vi "HFRR ADV v04.vi"() -> ()   [LabVIEW 2025] (continued)
              n1811 = String Subset(string=w2060, offset (0)=35, length (rest)=9 ("length (rest)")) -> (substring=w2085:string)
              n1812 = String Subset(string=w2060, offset (0)=55, length (rest)=9 ("length (rest)")) -> (substring=w2071:string)
              n1813 = String Subset(string=w2060, offset (0)=25, length (rest)=9 ("length (rest)")) -> (substring=w2065:string)
              n1814 = String Subset(string=w2060, offset (0)=45, length (rest)=9 ("length (rest)")) -> (substring=w2073:string)
              n1815 = String Subset(string=w2060, offset (0)=0, length (rest)=14 ("length (rest)")) -> (substring=w2088:string)
              n1816 = String Subset(string=w2060, offset (0)=15, length (rest)=9 ("length (rest)")) -> (substring=w2091:string)
              n1817 = String Subset(string=w2060, offset (0)=65, length (rest)=9 ("length (rest)")) -> (substring=w2077:string)
              n1818 = Fract/Exp String To Number(string=w2063) -> (number=w2059:dbl)  [unwired: 3 in, 1 out]
              n1819 = Fract/Exp String To Number(string=w2085) -> (number=w2083:dbl)  [unwired: 3 in, 1 out]
              n1820 = Fract/Exp String To Number(string=w2071) -> (number=w2068:dbl)  [unwired: 3 in, 1 out]
              n1821 = Fract/Exp String To Number(string=w2065) -> (number=w2064:dbl)  [unwired: 3 in, 1 out]
              n1822 = Fract/Exp String To Number(string=w2073) -> (number=w2072:dbl)  [unwired: 3 in, 1 out]
              n1823 = Fract/Exp String To Number(string=w2088) -> (number=w2084:dbl)  [unwired: 3 in, 1 out]
              n1824 = Fract/Exp String To Number(string=w2091) -> (number=w2082:dbl)  [unwired: 3 in, 1 out]
              n1825 = Fract/Exp String To Number(string=w2077) -> (number=w2080:dbl)  [unwired: 3 in, 1 out]
              n1826 = Add(x=w2080, y=0.0) -> (x+y=w2076:dbl)
            }
            n1827 = for {
              N: w1968 -> [_]
              tunnel: w1975 -> [w2023]
              tunnel: w1974 -> [w2022]
              tunnel: [w2012] -> w1928 mode=indexing
              tunnel: [w2011] -> w1921 mode=indexing
              tunnel: w1965 -> [_]
              tunnel: [w2000] -> w1926 mode=indexing
              tunnel: [w2005] -> w1923 mode=indexing
              tunnel: [w2001] -> w1913 mode=indexing
              tunnel: [w1996] -> w1888 mode=indexing
              tunnel: [w1992] -> w1869 mode=indexing
              tunnel: [w1987] -> w1829 mode=indexing
              (unwired) 1.0 ("x")
              (unwired) TRUE ("line mode (F)")
              n1828 = Read from Text File "Read File"(file (use dialog)=w2023, error in=w2022) -> (text=w1988:string)  [unwired: 2 in, 3 out]
              n1829 = local write "String 12"(w1988) -> ()
              n1830 = String Subset(string=w1988, offset (0)=85, length (rest)=9 ("length (rest)")) -> (substring=w1990:string)
              n1831 = String Subset(string=w1988, offset (0)=35, length (rest)=9 ("length (rest)")) -> (substring=w2013:string)
              n1832 = String Subset(string=w1988, offset (0)=55, length (rest)=9 ("length (rest)")) -> (substring=w1998:string)
              n1833 = String Subset(string=w1988, offset (0)=25, length (rest)=9 ("length (rest)")) -> (substring=w1994:string)
              n1834 = String Subset(string=w1988, offset (0)=45, length (rest)=9 ("length (rest)")) -> (substring=w2003:string)
              n1835 = String Subset(string=w1988, offset (0)=15, length (rest)=9 ("length (rest)")) -> (substring=w2019:string)
              n1836 = String Subset(string=w1988, offset (0)=0, length (rest)=14 ("length (rest)")) -> (substring=w2016:string)
              n1837 = String Subset(string=w1988, offset (0)=65, length (rest)=9 ("length (rest)")) -> (substring=w2006:string)
              n1838 = Fract/Exp String To Number(string=w1990) -> (number=w1987:dbl)  [unwired: 3 in, 1 out]
              n1839 = Fract/Exp String To Number(string=w2013) -> (number=w2011:dbl)  [unwired: 3 in, 1 out]
              n1840 = Fract/Exp String To Number(string=w1998) -> (number=w1996:dbl)  [unwired: 3 in, 1 out]
              n1841 = Fract/Exp String To Number(string=w1994) -> (number=w1992:dbl)  [unwired: 3 in, 1 out]
              n1842 = Fract/Exp String To Number(string=w2003) -> (number=w2001:dbl)  [unwired: 3 in, 1 out]
              n1843 = Fract/Exp String To Number(string=w2019) -> (number=w2000:dbl)  [unwired: 3 in, 1 out]
              n1844 = Fract/Exp String To Number(string=w2016) -> (number=w2012:dbl)  [unwired: 3 in, 1 out]
              n1845 = Fract/Exp String To Number(string=w2006) -> (number=w2009:dbl)  [unwired: 3 in, 1 out]
              n1846 = Add(x=w2009, y=0.0) -> (x+y=w2005:dbl)
            }
            n1847 = Delete From Array(array=w1871, index=0) -> (array with subset deleted=w1844:dbl[])  [unwired: 1 in, 1 out]
            n1848 = Delete From Array(array=w1934, index=0) -> (array with subset deleted=w1907:dbl[])  [unwired: 1 in, 1 out]
            n1849 = Delete From Array(array=w1914, index=0) -> (array with subset deleted=w1902:dbl[])  [unwired: 1 in, 1 out]
            n1850 = Delete From Array(array=w1932, index=0) -> (array with subset deleted=w1933:dbl[])  [unwired: 1 in, 1 out]
            n1851 = call-poly <vilib>:"Mean.vi"("X"=w1844) -> ("mean"=→"КОФ2 4":dbl)  [unwired: 1 out]
            n1852 = call-poly <vilib>:"Mean.vi"("X"=w1907) -> ("mean"=→"КОФ3":dbl)  [unwired: 1 out]
            n1853 = call-poly <vilib>:"Mean.vi"("X"=w1902) -> ("mean"=→"CP3":dbl)  [unwired: 1 out]
            n1854 = Delete From Array(array=w1896, index=0) -> (array with subset deleted=w1823:dbl[])  [unwired: 1 in, 1 out]
            n1855 = Delete From Array(array=w1835, index=0) -> (array with subset deleted=w1822:dbl[])  [unwired: 1 in, 1 out]
            n1856 = Delete From Array(array=w1875, index=0) -> (array with subset deleted=w1846:dbl[])  [unwired: 1 in, 1 out]
            n1857 = Delete From Array(array=w1953, index=0) -> (array with subset deleted=w1908:dbl[])  [unwired: 1 in, 1 out]
            n1858 = Delete From Array(array=w1919, index=0) -> (array with subset deleted=w1904:dbl[])  [unwired: 1 in, 1 out]
            "array w/ subset deleted" <- w1904
            n1859 = Delete From Array(array=w1950, index=0) -> (array with subset deleted=w1951:dbl[])  [unwired: 1 in, 1 out]
            n1860 = call-poly <vilib>:"Mean.vi"("X"=w1846) -> ("mean"=→"КОФ2 2":dbl)  [unwired: 1 out]
            n1861 = call-poly <vilib>:"Mean.vi"("X"=w1908) -> ("mean"=→"КОФ1":dbl)  [unwired: 1 out]
            n1862 = Bundle "Bundle"(w1823, w1822) -> (w1828:cluster{dbl[], dbl[]})  [unwired: 1 in]
            n1863 = Bundle "Bundle"(w1823, w1951) -> (w1815:cluster{dbl[], dbl[]})  [unwired: 1 in]
            n1864 = Delete From Array(array=w1830, index=0) -> (array with subset deleted=w1818:dbl[])  [unwired: 1 in, 1 out]
            n1865 = Delete From Array(array=w1831, index=0) -> (array with subset deleted=w1820:dbl[])  [unwired: 1 in, 1 out]
            n1866 = Delete From Array(array=w1941, index=0) -> (array with subset deleted=w1942:dbl[])  [unwired: 1 in, 1 out]
            n1867 = Delete From Array(array=w1829, index=0) -> (array with subset deleted=w1816:dbl[])  [unwired: 1 in, 1 out]
            n1868 = Delete From Array(array=w1923, index=0) -> (array with subset deleted=w1924:dbl[])  [unwired: 1 in, 1 out]
            n1869 = Delete From Array(array=w1948, index=0) -> (array with subset deleted=w1854:dbl[])  [unwired: 1 in, 1 out]
            n1870 = Delete From Array(array=w1894, index=0) -> (array with subset deleted=w1850:dbl[])  [unwired: 1 in, 1 out]
            n1871 = Delete From Array(array=w1930, index=0) -> (array with subset deleted=w1852:dbl[])  [unwired: 1 in, 1 out]
            n1872 = Delete From Array(array=w1890, index=0) -> (array with subset deleted=w1848:dbl[])  [unwired: 1 in, 1 out]
            n1873 = Delete From Array(array=w1939, index=0) -> (array with subset deleted=w1853:dbl[])  [unwired: 1 in, 1 out]
            n1874 = Delete From Array(array=w1892, index=0) -> (array with subset deleted=w1849:dbl[])  [unwired: 1 in, 1 out]
            n1875 = Delete From Array(array=w1873, index=0) -> (array with subset deleted=w1845:dbl[])  [unwired: 1 in, 1 out]
            n1876 = Delete From Array(array=w1917, index=0) -> (array with subset deleted=w1903:dbl[])  [unwired: 1 in, 1 out]
            n1877 = Delete From Array(array=w1944, index=0) -> (array with subset deleted=w1905:dbl[])  [unwired: 1 in, 1 out]
            n1878 = Delete From Array(array=w1921, index=0) -> (array with subset deleted=w1851:dbl[])  [unwired: 1 in, 1 out]
            n1879 = Delete From Array(array=w1888, index=0) -> (array with subset deleted=w1847:dbl[])  [unwired: 1 in, 1 out]
            n1880 = Delete From Array(array=w1869, index=0) -> (array with subset deleted=w1843:dbl[])  [unwired: 1 in, 1 out]
            n1881 = Delete From Array(array=w1913, index=0) -> (array with subset deleted=w1901:dbl[])  [unwired: 1 in, 1 out]
            n1882 = Delete From Array(array=w1926, index=0) -> (array with subset deleted=w1906:dbl[])  [unwired: 1 in, 1 out]
            n1883 = Delete From Array(array=w1936, index=0) -> (array with subset deleted=w1819:dbl[])  [unwired: 1 in, 1 out]
            n1884 = Delete From Array(array=w1946, index=0) -> (array with subset deleted=w1821:dbl[])  [unwired: 1 in, 1 out]
            n1885 = Delete From Array(array=w1928, index=0) -> (array with subset deleted=w1817:dbl[])  [unwired: 1 in, 1 out]
            n1886 = Bundle "Bundle"(w1823, w1854) -> (w1841:cluster{dbl[], dbl[]})  [unwired: 1 in]
            n1887 = Bundle "Bundle"(w1823, w1908) -> (w1842:cluster{dbl[], dbl[]})  [unwired: 1 in]
            n1888 = Bundle "Bundle"(w1854, w1850) -> (w1856:cluster{dbl[], dbl[]})  [unwired: 1 in]
            n1889 = Bundle "Bundle"(w1819, w1818) -> (w1826:cluster{dbl[], dbl[]})  [unwired: 1 in]
            n1890 = Bundle "Bundle"(w1852, w1848) -> (w1858:cluster{dbl[], dbl[]})  [unwired: 1 in]
            n1891 = Bundle "Bundle"(w1819, w1852) -> (w1962:cluster{dbl[], dbl[]})  [unwired: 1 in]
            n1892 = Bundle "Bundle"(w1819, w1848) -> (w1886:cluster{dbl[], dbl[]})  [unwired: 1 in]
            n1893 = Bundle "Bundle"(w1819, w1907) -> (w1972:cluster{dbl[], dbl[]})  [unwired: 1 in]
            n1894 = Bundle "Bundle"(w1819, w1902) -> (w1910:cluster{dbl[], dbl[]})  [unwired: 1 in]
            n1895 = Bundle "Bundle"(w1819, w1933) -> (w1957:cluster{dbl[], dbl[]})  [unwired: 1 in]
            n1896 = Bundle "Bundle"(w1853, w1849) -> (w1857:cluster{dbl[], dbl[]})  [unwired: 1 in]
            n1897 = Bundle "Bundle"(w1821, w1820) -> (w1827:cluster{dbl[], dbl[]})  [unwired: 1 in]
            n1898 = Bundle "Bundle"(w1821, w1853) -> (w1964:cluster{dbl[], dbl[]})  [unwired: 1 in]
            n1899 = Bundle "Bundle"(w1821, w1849) -> (w1887:cluster{dbl[], dbl[]})  [unwired: 1 in]
            n1900 = Bundle "Bundle"(w1821, w1903) -> (w1911:cluster{dbl[], dbl[]})  [unwired: 1 in]
            n1901 = Bundle "Bundle"(w1821, w1905) -> (w1973:cluster{dbl[], dbl[]})  [unwired: 1 in]
            n1902 = Bundle "Bundle"(w1821, w1942) -> (w1955:cluster{dbl[], dbl[]})  [unwired: 1 in]
            n1903 = Bundle "Bundle"(w1851, w1847) -> (w1859:cluster{dbl[], dbl[]})  [unwired: 1 in]
            n1904 = Bundle "Bundle"(w1817, w1816) -> (w1825:cluster{dbl[], dbl[]})  [unwired: 1 in]
            n1905 = Bundle "Bundle"(w1817, w1851) -> (w1963:cluster{dbl[], dbl[]})  [unwired: 1 in]
            n1906 = Bundle "Bundle"(w1817, w1847) -> (w1885:cluster{dbl[], dbl[]})  [unwired: 1 in]
            n1907 = Bundle "Bundle"(w1817, w1901) -> (w1909:cluster{dbl[], dbl[]})  [unwired: 1 in]
            n1908 = Bundle "Bundle"(w1817, w1906) -> (w1971:cluster{dbl[], dbl[]})  [unwired: 1 in]
            n1909 = Bundle "Bundle"(w1817, w1924) -> (w1956:cluster{dbl[], dbl[]})  [unwired: 1 in]
            n1910 = call-poly <vilib>:"Mean.vi"("X"=w1904) -> ("mean"=→"CP1":dbl)  [unwired: 1 out]
            n1911 = call-poly <vilib>:"Mean.vi"("X"=w1845) -> ("mean"=→"КОФ2 3":dbl)  [unwired: 1 out]
            n1912 = call-poly <vilib>:"Mean.vi"("X"=w1903) -> ("mean"=→"CP2":dbl)  [unwired: 1 out]
            n1913 = call-poly <vilib>:"Mean.vi"("X"=w1905) -> ("mean"=→"КОФ2":dbl)  [unwired: 1 out]
            n1914 = call-poly <vilib>:"Mean.vi"("X"=w1843) -> ("mean"=→"КОФ2 5":dbl)  [unwired: 1 out]
            n1915 = call-poly <vilib>:"Mean.vi"("X"=w1901) -> ("mean"=→"CP4":dbl)  [unwired: 1 out]
            n1916 = call-poly <vilib>:"Mean.vi"("X"=w1906) -> ("mean"=→"КОФ4":dbl)  [unwired: 1 out]
            n1917 = Bundle "Bundle"(w1823, w1850) -> (w1814:cluster{dbl[], dbl[]})  [unwired: 1 in]
            n1918 = Bundle "Bundle"(w1823, w1904) -> (w1837:cluster{dbl[], dbl[]})  [unwired: 1 in]
            n1919 = Build Array "Build Array"(w1814, w1837) -> (w1840:cluster{dbl[], dbl[]}[])
            "XY Graph 17" <- w1840
            n1920 = Build Array "Build Array"(w1828, w1827, w1826, w1825) -> (→"Frequency ( Hz )":cluster{dbl[], dbl[]}[])
            n1921 = Build Array "Build Array"(w1856, w1857, w1858, w1859) -> (→"Air Temp ( °C ) vs Humidity ( % RH )":cluster{dbl[], dbl[]}[])
            n1922 = Build Array "Build Array"(w1841, w1964, w1962, w1963) -> (→"Air Temperature  ( °C )":cluster{dbl[], dbl[]}[])
            n1923 = Build Array "Build Array"(w1814, w1887, w1886, w1885) -> (→"Humidity ( %RH )":cluster{dbl[], dbl[]}[])
            n1924 = Build Array "Build Array"(w1842, w1973, w1972, w1971) -> (→"Coefficient Of Friction":cluster{dbl[], dbl[]}[])
            n1925 = Build Array "Build Array"(w1837, w1911, w1910, w1909) -> (→"Sample Temperature ( °C )":cluster{dbl[], dbl[]}[])
            n1926 = Build Array "Build Array"(w1815, w1955, w1957, w1956) -> (→"XY Graph 13":cluster{dbl[], dbl[]}[])
            n1927 = Bundle "Bundle"(w1823, w1846) -> (w1868:cluster{dbl[], dbl[]})  [unwired: 1 in]
            n1928 = Bundle "Bundle"(w1819, w1844) -> (w1866:cluster{dbl[], dbl[]})  [unwired: 1 in]
            n1929 = Bundle "Bundle"(w1821, w1845) -> (w1867:cluster{dbl[], dbl[]})  [unwired: 1 in]
            n1930 = Bundle "Bundle"(w1817, w1843) -> (w1865:cluster{dbl[], dbl[]})  [unwired: 1 in]
            n1931 = Build Array "Build Array"(w1868, w1867, w1866, w1865) -> (→"Stroke ( mm )":cluster{dbl[], dbl[]}[])
            n1932 = local write "XY Graph 16"(w1840) -> ()
          }
          frame #2 {
          }
          frame #3 {
            n1933 = local write "Numeric 8"(0 ("Numeric 8")) -> ()
            n1934 = local write "Numeric 11"(0 ("Numeric 11")) -> ()
            n1935 = local write "Numeric 12"(0 ("Numeric 12")) -> ()
            n1936 = local write "Numeric 13"(0 ("Numeric 13")) -> ()
            n1937 = property on="OPEN" class="Bool (strict)"("Visible"=TRUE) -> ()  [unwired: 2 in, 2 out]
            n1938 = local read "String Control 2"() -> (w2140:string)
            n1939 = local read "String Control 4"() -> (w2139:string)
            n1940 = local read "String Control 6"() -> (w2138:string)
            n1941 = local read "String Control 8"() -> (w2137:string)
            n1942 = Match Pattern(string=w2140, regular expression="Samples / cycle :- ") -> (after substring=w2154:string)  [unwired: 1 in, 3 out]
            n1943 = Match Pattern(string=w2140, regular expression="Frequency :- ") -> (after substring=w2173:string)  [unwired: 1 in, 3 out]
            n1944 = Match Pattern(string=w2139, regular expression="Samples / cycle :- ") -> (after substring=w2150:string)  [unwired: 1 in, 3 out]
            n1945 = Match Pattern(string=w2139, regular expression="Frequency :- ") -> (after substring=w2168:string)  [unwired: 1 in, 3 out]
            n1946 = Match Pattern(string=w2138, regular expression="Samples / cycle :- ") -> (after substring=w2146:string)  [unwired: 1 in, 3 out]
            n1947 = Match Pattern(string=w2138, regular expression="Frequency :- ") -> (after substring=w2163:string)  [unwired: 1 in, 3 out]
            n1948 = Match Pattern(string=w2137, regular expression="Samples / cycle :- ") -> (after substring=w2142:string)  [unwired: 1 in, 3 out]
            n1949 = Match Pattern(string=w2137, regular expression="Frequency :- ") -> (after substring=w2158:string)  [unwired: 1 in, 3 out]
            n1950 = String Subset(string=w2154, length (rest)=6 ("length (rest)")) -> (substring=w2156:string)  [unwired: 1 in]
            n1951 = String Subset(string=w2173, length (rest)=9 ("length (rest)")) -> (substring=w2175:string)  [unwired: 1 in]
            n1952 = String Subset(string=w2150, length (rest)=6 ("length (rest)")) -> (substring=w2152:string)  [unwired: 1 in]
            n1953 = String Subset(string=w2168, length (rest)=9 ("length (rest)")) -> (substring=w2170:string)  [unwired: 1 in]
            n1954 = String Subset(string=w2146, length (rest)=6 ("length (rest)")) -> (substring=w2148:string)  [unwired: 1 in]
            n1955 = String Subset(string=w2163, length (rest)=9 ("length (rest)")) -> (substring=w2165:string)  [unwired: 1 in]
            n1956 = String Subset(string=w2142, length (rest)=6 ("length (rest)")) -> (substring=w2144:string)  [unwired: 1 in]
            n1957 = String Subset(string=w2158, length (rest)=9 ("length (rest)")) -> (substring=w2160:string)  [unwired: 1 in]
            n1958 = Fract/Exp String To Number(string=w2156) -> (number=w2136:dbl)  [unwired: 3 in, 1 out]
            n1959 = Fract/Exp String To Number(string=w2175) -> (number=w2176:dbl)  [unwired: 3 in, 1 out]
            n1960 = Fract/Exp String To Number(string=w2152) -> (number=w2135:dbl)  [unwired: 3 in, 1 out]
            n1961 = Fract/Exp String To Number(string=w2170) -> (number=w2171:dbl)  [unwired: 3 in, 1 out]
            n1962 = Fract/Exp String To Number(string=w2148) -> (number=w2134:dbl)  [unwired: 3 in, 1 out]
            n1963 = Fract/Exp String To Number(string=w2165) -> (number=w2166:dbl)  [unwired: 3 in, 1 out]
            n1964 = Fract/Exp String To Number(string=w2144) -> (number=w2133:dbl)  [unwired: 3 in, 1 out]
            n1965 = Fract/Exp String To Number(string=w2160) -> (number=w2161:dbl)  [unwired: 3 in, 1 out]
            n1966 = local write "sample1"(w2136) -> ()
            n1967 = local write "freq1"(w2176) -> ()
            n1968 = local write "sample2"(w2135) -> ()
            n1969 = local write "freq2"(w2171) -> ()
            n1970 = local write "sample3"(w2134) -> ()
            n1971 = local write "freq3"(w2166) -> ()
            n1972 = local write "sample4"(w2133) -> ()
            n1973 = local write "freq 4"(w2161) -> ()
          }
        }
      }
    }
    n1974 = case shown="True" w1625 {
      selector: w1625 -> [_ w1753]
      frame False {
      }
      frame True {
        n1975 = Not(x=w1753) -> (.not. x?=w1749:bool)
        n1976 = local write "service 3"(w1749) -> ()
        n1977 = local write "OPEN 6"(w1749) -> ()
        n1978 = call <vilib>:"System Exec.vi"("wait until completion? (T)"=TRUE, "command line"="C:\\LAB-IQ\\Scar View.exe") -> ("error out"=→"error out 5":errorcluster)  [unwired: 6 in, 3 out]
      }
    }
    n1979 = case shown="\"Acquire\", Default" w1636 {
      frame "Acquire", Default {
        w2649 = 0.2 ("y")
        w2654 = 1.0 ("y")
        w2655 = 0.8 ("y")
        # "Elapsed time\ncof\nstroke\nAir temp\nTemp\nHumidity"
        n1980 = disable-structure shown="Disabled" {
          frame Disabled {
            n1981 = local read "Flag"() -> (w2672:dbl)
            n1982 = local read "RUN"() -> (w2669:bool)
            n1983 = Not(x=w2669) -> (.not. x?=w2668:bool)
            n1984 = Equal?(x=w2672, y=10.0) -> (x = y?=w2670:bool)
            n1985 = And(x=w2670, y=w2668) -> (x .and. y?=w2667:bool)
            n1986 = case shown="True" w2667 {
              frame False {
              }
              frame True {
                w2673 = FALSE ("Heater Button")
                n1987 = local write "Humidity"(w2673) -> ()
                n1988 = local write "Heater Button"(w2673) -> ()
              }
            }
          }
          frame Enabled {
          }
        }
        n1989 = disable-structure shown="Disabled" {
          frame Disabled {
            n1990 = case shown="True" {
              selector: _ -> [_ _]
              frame False {
              }
              frame True {
                w2764 = TRUE ("Heater")
                n1991 = local write "Humidity"(w2764) -> ()
                n1992 = local write "Heater Button"(w2764) -> ()
                n1993 = local read "TEST STANDARD"() -> (w2767:T3)
                n1994 = local read "TEST STANDARD"() -> (w2762:T3)
                n1995 = Equal?(x=w2767, y=enum16{"ASTM D6079", "ISO 12156", "Custom"}."ISO 12156" ("Test Standard")) -> (x = y?=w2765:bool)
                n1996 = Equal?(x=w2762, y=enum16{"ASTM D6079", "ISO 12156", "Custom"}."ASTM D6079" ("Test Standard")) -> (x = y?=w2761:bool)
                n1997 = case shown="True" w2765 {
                  frame False {
                  }
                  frame True {
                    n1998 = local write "Heater"(TRUE ("Heater")) -> ()
                    n1999 = local write "airtempflg"(FALSE ("airtempflg")) -> ()
                  }
                }
                n2000 = case shown="True" w2761 {
                  frame False {
                  }
                  frame True {
                    n2001 = local write "Heater"(FALSE ("Heater")) -> ()
                    n2002 = local write "airtempflg"(TRUE ("airtempflg")) -> ()
                  }
                }
              }
            }
          }
          frame Enabled {
          }
        }
        n2003 = stacked-sequence {
          frame #0 {
            n2004 = case shown="True" "RST FF" {
              frame False {
              }
              frame True {
                w2830 = 0.0 ("X Scale.Range:Maximum")
                n2005 = property on="Frictional Force ( N )" class="WFChart (strict)"("XScale.Maximum"=600.0 ("X Scale.Range:Maximum"), "XScale.Minimum"=w2830, "YScale.Maximum"=10.0 ("Y Scale.Range:Maximum"), "YScale.Minimum"=w2830) -> ()  [unwired: 2 in, 2 out]
              }
            }
          }
          frame #1 {
            n2006 = case shown="True" "RST TEMP" {
              frame False {
              }
              frame True {
                n2007 = property on="Temperature ( Deg C )" class="WFChart (strict)"("XScale.Minimum"=0.0 ("X Scale.Range:Minimum"), "XScale.Maximum"=600.0 ("X Scale.Range:Maximum"), "YScale.Minimum"=0.0 ("Y Scale.Range:Minimum"), "YScale.Maximum"=100.0 ("Y Scale.Range:Maximum")) -> ()  [unwired: 2 in, 2 out]
              }
            }
          }
          frame #2 {
            n2008 = case shown="True" "RSTCOF" {
              frame False {
              }
              frame True {
                n2009 = property on="Coefficient of Friction" class="WFChart (strict)"("XScale.Minimum"=0.0 ("X Scale.Range:Minimum"), "XScale.Maximum"=600.0 ("X Scale.Range:Maximum"), "YScale.Maximum"=1.0 ("X Scale.Range:Minimum"), "YScale.Minimum"=0.0 ("X Scale.Range:Minimum")) -> ()  [unwired: 2 in, 2 out]
              }
            }
          }
          frame #3 {
            n2010 = case shown="True" "RSTCOF 2" {
              frame False {
              }
              frame True {
                (unwired) 100.0 ("Y Scale.Range:Maximum")
                (unwired) 0.0 ("Y Scale.Range:Minimum")
                (unwired) 600.0 ("X Scale.Range:Maximum")
                (unwired) 0.0 ("X Scale.Range:Minimum")
              }
            }
          }
          frame #4 {
            n2011 = case shown="True" "RSTCOF 3" {
              frame False {
              }
              frame True {
                n2012 = property on="Electrical Contact Resistance ( % )" class="WFChart (strict)"("XScale.Minimum"=0.0 ("X Scale.Range:Minimum"), "XScale.Maximum"=600.0 ("X Scale.Range:Maximum"), "YScale.Minimum"=0.0 ("Y Scale.Range:Minimum"), "YScale.Maximum"=100.0 ("Y Scale.Range:Maximum")) -> ()  [unwired: 2 in, 2 out]
              }
            }
          }
        }
        n2013 = disable-structure shown="Disabled" {
          frame Disabled {
            n2014 = case shown="True" {
              selector: _ -> [_ _]
              frame False {
              }
              frame True {
                n2015 = local read "zflag 2"() -> (w2731:dbl)
                n2016 = local read "yflag"() -> (w2733:dbl)
                n2017 = Equal?(x=w2733, y=2.0 ("tflag")) -> (x = y?=w2735:bool)
                n2018 = Equal?(x=w2731, y=3.0 ("tflag")) -> (x = y?=w2734:bool)
                n2019 = And(x=w2735, y=w2734) -> (x .and. y?=w2729:bool)
                n2020 = case shown="True" w2729 {
                  frame False {
                  }
                  frame True {
                    w2760 = 0.0 ("zflag")
                    n2021 = local write "zflag"(w2760) -> ()
                    n2022 = local write "zflag 2"(w2760) -> ()
                    n2023 = Delete(path (use dialog)=path "C:/LAB-IQ-NXT/WO 2449 TT.sig" ("file path (dialog if empty)")) -> (deleted path=w2759:path)  [unwired: 4 in, 2 out]
                    n2024 = Delete(path (use dialog)=path "C:/LAB-IQ-NXT/WO 2449 TRH.sig" ("file path (dialog if empty)")) -> (deleted path=w2754:path)  [unwired: 4 in, 2 out]
                    n2025 = local read "SEN.RUN HRS"() -> (w2746:dbl)
                    n2026 = local read "SENSOR TIME"() -> (w2744:dbl)
                    n2027 = call <vilib>:"compatOverwrite.vi"("overwrite (F)"=TRUE) -> ("overwrite?"=w2736:T23)
                    n2028 = call <vilib>:"compatOverwrite.vi"("overwrite (F)"=TRUE) -> ("overwrite?"=w2740:T23)
                    n2029 = local read "Total No. of Tests"() -> (w2747:dbl)
                    n2030 = Add(x=w2744, y=w2746) -> (x+y=w2745:dbl)
                    "SEN.RUN HRS" <- w2745
                    n2031 = Open/Create/Replace File(file path (use dialog)=w2759, operation (0:open)=w2736) -> (refnum out=w2737:refnum<file>, error out=w2738:errorcluster)  [unwired: 4 in, 1 out]
                    n2032 = Open/Create/Replace File(file path (use dialog)=w2754, operation (0:open)=w2740) -> (refnum out=w2741:refnum<file>, error out=w2742:errorcluster)  [unwired: 4 in, 1 out]
                    n2033 = Deny Access(4:w2738, 6:T21."deny none" ("deny mode (2)"), 7:w2737) -> (3:w2758:refnum<file>)  [unwired: 1 out]
                    n2034 = Deny Access(4:w2742, 6:T21."deny none" ("deny mode (2)"), 7:w2741) -> (3:w2750:refnum<file>)  [unwired: 1 out]
                    n2035 = Number To Decimal String(number=w2747) -> (decimal integer string=w2755:string)  [unwired: 1 in]
                    n2036 = Number To Decimal String(number=w2745) -> (decimal integer string=w2751:string)  [unwired: 1 in]
                    n2037 = Write to Binary File(file (use dialog)=w2758, data=w2755, 5:FALSE ("prepend array or string size? (T)")) -> ()  [unwired: 3 in, 3 out]
                    n2038 = Write to Binary File(file (use dialog)=w2750, data=w2751, 5:FALSE ("prepend array or string size? (T)")) -> ()  [unwired: 3 in, 3 out]
                  }
                }
              }
            }
          }
          frame Enabled {
          }
        }
        n2039 = local read "RUN"() -> (w2658:bool)
        n2040 = local read "run replace"() -> (w2662:bool)
        n2041 = local read "run replace"() -> (w2661:bool)
        n2042 = case shown="True" w2658 {
          frame False {
            n2043 = local write "run replace"(FALSE ("run replace")) -> ()
          }
          frame True {
            "run replace" <- TRUE ("run replace")
          }
        }
        n2044 = local read "RUN"() -> (w2666:bool)
        n2045 = local read "Set Temp"() -> (w2628:dbl)
        n2046 = local read "SetTemp"() -> (w2630:dbl)
        n2047 = case shown="False" w2666 {
          tunnel: [FALSE ("TEST RUNNING") TRUE ("TEST RUNNING")] -> w2665
          frame False {
            w2849 = 0.0 ("Flag")
            n2048 = local write "Elapsed time"(0.0 ("elapsedtime")) -> ()
            n2049 = local write "Time Remaining"(w2849) -> ()
            n2050 = local write "Flag"(w2849) -> ()
            n2051 = local write "Remaining Time"(w2849) -> ()
          }
          frame True {
            n2052 = local write "Flag"(10.0 ("Flag")) -> ()
          }
        }
        n2053 = case shown="False" w2662 {
          frame False {
            n2054 = local read "zflag"() -> (→"zflag 2":dbl)
            n2055 = local write "yflag"(2.0 ("tflag")) -> ()
            n2056 = local write "FLAG 4"(0.0 ("FLAG")) -> ()
          }
          frame True {
            n2057 = local write "yflag"(1.0 ("tflag")) -> ()
            n2058 = local write "zflag"(3.0 ("zflag")) -> ()
          }
        }
        n2059 = local read "acq 2"() -> (w2660:bool)
        n2060 = local read "AIR TEMP"() -> (w2623:dbl)
        n2061 = local read "Amb temp"() -> (w2627:dbl)
        n2062 = case shown="True" "Save & Continue" {
          frame False {
          }
          frame True {
            "acq 2" <- TRUE ("acq 2")
          }
        }
        n2063 = local read "Set Rh"() -> (w2629:dbl)
        n2064 = Add(x=w2630, y=w2655) -> (x+y=w2656:dbl)
        n2065 = Subtract(x=w2630, y=w2655) -> (x-y=w2657:dbl)
        n2066 = Add(x=w2628, y=w2649) -> (x+y=w2650:dbl)
        n2067 = Subtract(x=w2628, y=w2649) -> (x-y=w2651:dbl)
        n2068 = And(x=w2660, y=w2661) -> (x .and. y?=w2659:bool)
        n2069 = Greater Or Equal?(x=w2623, y=15.0) -> (x >= y?=w2624:bool)
        "powstat" <- w2624
        n2070 = local read "Humidity ( %RH )"() -> (w2626:dbl)
        n2071 = case shown="True" "Save & Continue" {
          frame False {
          }
          frame True {
            n2072 = while {
              tunnel: "0123456789abcdefghijklmnopqrstuvwxyzABCDEFGHIJKLMNOPQRSTUVWXYZ" ("string 2") -> [w2820]
              shift-right: [w2818] -> w2813
              shift-left: "" -> [w2817]
              i -> [w2827]
              stop <- w2826 stop-if-true
              n2073 = Random Number (0-1)() -> (number: 0 to 1=w2821:dbl)
              n2074 = Multiply(x=w2821, y=62.0) -> (x*y=w2823:dbl)
              n2075 = Decrement(x="Length") -> (x-1=w2816:i16)
              n2076 = To Word Integer(number=w2823) -> (16bit integer=w2824:i16)
              n2077 = String Subset(string=w2820, offset (0)=w2824, length (rest)=1 ("length (rest)")) -> (substring=w2819:string)
              n2078 = Greater Or Equal?(x=w2827, y=w2816) -> (x >= y?=w2826:bool)
              n2079 = Concatenate Strings(w2819, w2817) -> (w2818:string)
            }
            n2080 = local write "UUID"(w2813) -> ()
          }
        }
        n2081 = In Range and Coerce(upper limit=w2656, x=w2627, lower limit=w2657) -> (In Range?=w2646:bool)  [unwired: 1 out]
        n2082 = Add(x=w2629, y=w2654) -> (x+y=w2653:dbl)
        n2083 = Subtract(x=w2629, y=w2654) -> (x-y=w2652:dbl)
        n2084 = local read "TEMP"() -> (w2625:dbl)
        n2085 = case shown="True" "Save & Continue" {
          frame False {
          }
          frame True {
            n2086 = local read "Operator ID"() -> (w3129:string)
            n2087 = local read "FILE"() -> (w3135:string)
            n2088 = String Length(string=w3135) -> (length=w3133:i32)
            n2089 = String Length(string=w3129) -> (length=w3130:i32)
            n2090 = Greater?(x=w3133, y=0) -> (0:w3132:bool)
            n2091 = Greater?(x=w3130, y=0) -> (0:w3128:bool)
            n2092 = And(x=w3132, y=w3128) -> (x .and. y?=w3127:bool)
            n2093 = case shown="True" w3127 {
              frame False {
                n2094 = stacked-sequence {
                  frame #0 {
                    n2095 = One Button Dialog(message="Please Enter a File Name and Operator ID to save data !", button name ("OK")="Ok") -> ()  [unwired: 1 out]
                  }
                  frame #1 {
                    n2096 = local write "Save & Continue"(FALSE ("OK Button")) -> ()
                  }
                }
                n2097 = local write "Save & Continue"(FALSE ("OK Button")) -> ()
              }
              frame True {
                n2098 = stacked-sequence {
                  frame #0 {
                    n2099 = local read "FILE"() -> (w3141:string)
                    n2100 = call "file check.vi"("file name in"=w3141) -> ("file name out"=w3140:string)  [unwired: 9 in, 1 out]
                    n2101 = call <vilib>:"Application Directory.vi"() -> ("Application Directory"=w3151:path)
                    n2102 = Build Path(base path=w3151, name or relative path="data") -> (appended path=w3150:path)
                    n2103 = call <vilib>:"Trim Whitespace.vi"("string"=w3140) -> ("trimmed string"=w3148:string)  [unwired: 1 in]
                    n2104 = call <vilib>:"Trim Whitespace.vi"("string"=w3140) -> ("trimmed string"=w3149:string)  [unwired: 1 in]
                    n2105 = List Folder(path=w3150) -> (folder names=w3146:string[])  [unwired: 3 in, 3 out]
                    n2106 = Match Pattern(string=w3148, regular expression="_(") -> (before substring=w3145:string)  [unwired: 1 in, 3 out]
                    n2107 = for {
                      tunnel: w3146 -> [w3160] mode=indexing
                      tunnel: w3145 -> [w3158]
                      shift-right: [w3156] -> w3143
                      shift-left: bool[] [] -> [w3157]
                      n2108 = Match Pattern(string=w3160, regular expression="_(") -> (before substring=w3159:string)  [unwired: 1 in, 3 out]
                      n2109 = Equal?(x=w3159, y=w3158) -> (x = y?=w3155:bool)
                      n2110 = case shown="True" w3155 {
                        tunnel: w3155 -> [_ w3163]
                        tunnel: w3157 -> [w3162 w3165]
                        tunnel: [w3162 w3164] -> w3156
                        frame False {
                        }
                        frame True {
                          n2111 = Insert Into Array(array=w3165, new element=w3163) -> (w3164:bool[])  [unwired: 1 in]
                        }
                      }
                    }
                    n2112 = Equal?(x=w3146, y=w3145) -> (x = y?=w3154:bool[])
                    n2113 = Or Array Elements(Boolean array=w3154) -> (logical OR=w3153:bool)
                    n2114 = Array Size(array=w3143) -> (size(s)=w3142:i32)
                    n2115 = case shown="True" w3153 {
                      tunnel: w3149 -> [_ w3173]
                      tunnel: w3142 -> [_ w3166]
                      frame False {
                      }
                      frame True {
                        n2116 = Number To Decimal String(number=w3166) -> (decimal integer string=w3169:string)  [unwired: 1 in]
                        n2117 = Search/Split String(string=w3173, search string/char (-)="_(" ("regular expression")) -> (substring before match=w3171:string)  [unwired: 1 in, 2 out]
                        n2118 = Concatenate Strings(w3171, "_(" ("regular expression"), w3169, ")" ("regular expression")) -> (w3167:string)
                        n2119 = local write "FILE"(w3167) -> ()
                      }
                    }
                  }
                  frame #1 {
                    w3175 = 0.0
                    w3188 = cluster{"y":dbl, dbl, "y":dbl}[] [] ("History Data")
                    w3189 = FALSE ("Heater Button")
                    (unwired) ")!" ("string")
                    (unwired) ")" ("string")
                    w3187 = dbl[] [] ("History Data")
                    w3193 = "\r"
                    # "C:\\WinDucom\\Data\\"
                    # "C:\\LAB-IQ-NXT\\data"
                    n2120 = local write "Humidity ( %RH )"(w3175) -> ()
                    n2121 = local write "Frequency ( Hz )"(w3175) -> ()
                    n2122 = local write "Stroke 3"(w3175) -> ()
                    n2123 = local write "speedop"(0.0 ("PIDclk 2")) -> ()
                    n2124 = local write "Set Temp 2"(65.0 ("Set Temp 2")) -> ()
                    n2125 = local write "AIR TEMP"(w3175) -> ()
                    n2126 = local write "clk"(0.0 ("clk")) -> ()
                    n2127 = local write "Stroke 4"(w3175) -> ()
                    n2128 = local write "COF 2"(w3175) -> ()
                    n2129 = local write "TEMP"(w3175) -> ()
                    n2130 = local write "ecr 3"(w3175) -> ()
                    n2131 = local write "FF 3"(w3175) -> ()
                    n2132 = local write "FF 2"(w3175) -> ()
                    n2133 = property on="Humidity ( %RH )" class="WFChart (strict)"("History Data"=w3187) -> ()  [unwired: 2 in, 2 out]
                    n2134 = property on="Coefficient of Friction" class="WFChart (strict)"("History Data"=w3187) -> ()  [unwired: 2 in, 2 out]
                    n2135 = property on="Coefficient of Friction" class="WFChart (strict)"("History Data"=w3187) -> ()  [unwired: 2 in, 2 out]
                    n2136 = property on="Frictional Force ( N )" class="WFChart (strict)"("History Data"=w3187) -> ()  [unwired: 2 in, 2 out]
                    n2137 = property on="Electrical Contact Resistance ( % )" class="WFChart (strict)"("History Data"=w3187) -> ()  [unwired: 2 in, 2 out]
                    n2138 = property on="Electrical Contact Resistance ( % )" class="WFChart (strict)"("History Data"=w3187) -> ()  [unwired: 2 in, 2 out]
                    n2139 = property on="Temperature ( Deg C )" class="WFChart (strict)"("History Data"=w3187) -> ()  [unwired: 2 in, 2 out]
                    n2140 = property on="Frictional Force ( N )" class="WFChart (strict)"("History Data"=w3187) -> ()  [unwired: 2 in, 2 out]
                    n2141 = property on="Coefficient of Friction" class="WFChart (strict)"("History Data"=w3187) -> ()  [unwired: 2 in, 2 out]
                    n2142 = property on="Frictional Force ( N )" class="WFChart (strict)"("History Data"=w3187) -> ()  [unwired: 2 in, 2 out]
                    n2143 = property on="Electrical Contact Resistance ( % )" class="WFChart (strict)"("History Data"=w3187) -> ()  [unwired: 2 in, 2 out]
                    n2144 = property on="Temperature ( Deg C )" class="WFChart (strict)"("History Data"=w3187) -> ()  [unwired: 2 in, 2 out]
                    n2145 = property on="Humidity ( %RH )" class="WFChart (strict)"("History Data"=w3187) -> ()  [unwired: 2 in, 2 out]
                    n2146 = property on="Stroke ( mm )" class="WFChart (strict)"("History Data"=w3188) -> ()  [unwired: 2 in, 2 out]
                    n2147 = property on="Stroke ( mm )" class="WFChart (strict)"("History Data"=w3188) -> ()  [unwired: 2 in, 2 out]
                    n2148 = local write "Humidity"(w3189) -> ()
                    n2149 = local write "Heater Button"(w3189) -> ()
                    n2150 = local read "FILE"() -> (w3183:string)
                    n2151 = disable-structure shown="Enabled" {
                      disable-tunnel: [w3228 _] -> w3174
                      frame Enabled {
                        n2152 = local read "NORMAL LOAD"() -> (w3228:dbl)
                      }
                      frame Disabled {
                      }
                    }
                    n2153 = call "file check.vi"("file name in"=w3183) -> ("error out"=w3186:errorcluster, "file name out"=w3180:string)  [unwired: 9 in]
                    n2154 = call "FILE PATH CREATION.vi"("error in"=w3186, "FILE NAME :"=w3180) -> ("FILE OUT"=w3179:path)  [unwired: 8 in, 1 out]
                    n2155 = Concatenate Strings(w3180, ".dgf" ("Substring")) -> (w3185:string)
                    n2156 = Concatenate Strings(w3180, ".duf" ("Substring")) -> (w3181:string)
                    n2157 = Multiply(x=w3174, y=1.0) -> (x*y=w3207:dbl)
                    n2158 = Build Path(base path=w3179, name or relative path=w3185) -> (appended path=w3178:path)
                    n2159 = Build Path(base path=w3179, name or relative path=w3181) -> (appended path=w3177:path)
                    n2160 = Number To Fractional String(number=w3207, width (-)=i16 5, precision (6)=i16 2) -> (F-format string=w3215:string)  [unwired: 1 in]
                    n2161 = local read "Fuel Discription :"() -> (w3203:string)
                    n2162 = local read "Batch Ref Num :"() -> (w3191:string)
                    n2163 = Get Date/Time String(date format (0)=enum16{"short", "long", "abbreviated"}."short") -> (date string=w3226:string, time string=w3223:string)  [unwired: 2 in]
                    n2164 = local read "Remarks :"() -> (w3202:string)
                    n2165 = Concatenate Strings("Load :- " ("Substring"), w3215, " grams ," ("Substring")) -> (w3214:string)
                    n2166 = local read "String 41"() -> (w3194:string)
                    n2167 = Concatenate Strings(w3203) -> (w3204:string)
                    n2168 = Concatenate Strings(w3191) -> (w3190:string)
                    n2169 = Concatenate Strings("tested by") -> (w3198:string)
                    n2170 = Concatenate Strings("(" ("Substring"), w3226, ")" ("Substring"), w3223) -> (w3196:string)
                    "concatenated string" <- w3196
                    n2171 = Concatenate Strings(w3202, "," ("string")) -> (w3201:string)
                    n2172 = Concatenate Strings("  TIME;      COF;       STROKE;     AIR TEMP;  TEMP;  HUMIDITY;  ECR; PID-OUT; FREQUENCY" ("Substring"), "\r") -> (w3210:string)
                    n2173 = Concatenate Strings(w3194, w3193, "Fuel Discription :-" ("Substring"), w3204, w3193, w3214, w3193, "Batch Ref Num :-" ("Substring"), w3190, w3193, " Remarks :- " ("Substring"), w3201, w3193, " Date :- " ("Substring"), w3196, w3193, "Tested By :-" ("Substring"), w3198) -> (w3208:string)
                    "REMARKS" <- w3208
                    n2174 = call <vilib>:"Write Characters To File.vi"("append to file? (new file:F)"=FALSE, "character string"=w3210, "file path (dialog if empty)"=w3178) -> ()  [unwired: 2 in, 1 out]
                    n2175 = call <vilib>:"Write Characters To File.vi"("append to file? (new file:F)"=FALSE, "character string"=w3208, "file path (dialog if empty)"=w3177) -> ()  [unwired: 2 in, 1 out]
                  }
                  frame #2 {
                    n2176 = local write "Cycles elapsed"(0 ("Cycles elapsed")) -> ()
                    n2177 = local write "cyclecount"(0 ("cyclecount")) -> ()
                    n2178 = local write "Save & Continue"(FALSE ("OK")) -> ()
                    n2179 = local write "autostrtflg"(TRUE ("autostrtflg")) -> ()
                    n2180 = local write "Save"(FALSE ("Save")) -> ()
                    n2181 = Get Date/Time In Seconds() -> (seconds since 1Jan1904=w3233:timestamp)
                    n2182 = To Double Precision Float(number=w3233) -> (double precision float=w3232:dbl)
                    n2183 = local write "acq timer"(w3232) -> ()
                    n2184 = One Button Dialog(message="Please ensure sample is mounted properly and machine is ready in all aspects for testing !", button name ("OK")="Ok") -> ()  [unwired: 1 out]
                  }
                  frame #3 {
                    n2185 = stacked-sequence {
                      frame #0 {
                        n2186 = local write "Main Dashboard Buttons"(T1."Dashboard" ("Main Dashboard Buttons")) -> ()
                        n2187 = local write "Main Tab"(T2."Acquire" ("Main Tab")) -> ()
                      }
                      frame #1 {
                        n2188 = local write "EVENT LOG"("" ("EVENT LOG")) -> ()
                      }
                      frame #2 {
                        n2189 = Wait (ms)(milliseconds to wait=u32 50) -> ()  [unwired: 1 out]
                      }
                      frame #3 {
                        n2190 = disable-structure shown="Disabled" {
                          frame Disabled {
                            n2191 = local read "EVENT LOG"() -> (w3245:string)
                            n2192 = call "Event Log.vi"("Content"="Test Details", "EVENT LOG"=w3245) -> ("EVENT LOG"=w3244:string)  [unwired: 8 in, 1 out]
                            n2193 = local write "EVENT LOG"(w3244) -> ()
                          }
                          frame Enabled {
                          }
                        }
                      }
                      frame #4 {
                        n2194 = Wait (ms)(milliseconds to wait=u32 50) -> ()  [unwired: 1 out]
                      }
                      frame #5 {
                        n2195 = local read "FILE"() -> (w3247:string)
                        n2196 = Concatenate Strings("File Name :" ("Content"), w3247) -> (w3248:string)
                        n2197 = local read "EVENT LOG"() -> (w3251:string)
                        n2198 = call "Event Log.vi"("Content"=w3248, "EVENT LOG"=w3251) -> ("EVENT LOG"=w3250:string)  [unwired: 8 in, 1 out]
                        n2199 = local write "EVENT LOG"(w3250) -> ()
                      }
                      frame #6 {
                        n2200 = Wait (ms)(milliseconds to wait=u32 50) -> ()  [unwired: 1 out]
                      }
                      frame #7 {
                        n2201 = local read "Batch Ref Num :"() -> (w3253:string)
                        n2202 = Concatenate Strings("Batch Ref No :" ("Content"), w3253) -> (w3254:string)
                        n2203 = local read "EVENT LOG"() -> (w3257:string)
                        n2204 = call "Event Log.vi"("Content"=w3254, "EVENT LOG"=w3257) -> ("EVENT LOG"=w3256:string)  [unwired: 8 in, 1 out]
                        n2205 = local write "EVENT LOG"(w3256) -> ()
                      }
                      frame #8 {
                        n2206 = Wait (ms)(milliseconds to wait=u32 50) -> ()  [unwired: 1 out]
                      }
                      frame #9 {
                        n2207 = local read "tested by"() -> (w3259:string)
                        n2208 = Concatenate Strings("Tested By :" ("Content"), w3259) -> (w3260:string)
                        n2209 = local read "EVENT LOG"() -> (w3263:string)
                        n2210 = call "Event Log.vi"("Content"=w3260, "EVENT LOG"=w3263) -> ("EVENT LOG"=w3262:string)  [unwired: 8 in, 1 out]
                        n2211 = local write "EVENT LOG"(w3262) -> ()
                      }
                      frame #10 {
                        n2212 = Wait (ms)(milliseconds to wait=u32 50) -> ()  [unwired: 1 out]
                      }
                      frame #11 {
                        n2213 = local read "TEST STANDARD"() -> (w3266:T3)
                        n2214 = case shown="\"ASTM D6079\", Default" w3266 {
                          tunnel: ["ASTM D6079" "ISO 12156" "CEC F-096-A-06" "Custom"] -> w3265
                          frame "ASTM D6079", Default {
                          }
                          frame "ISO 12156" {
                          }
                          frame "CEC F-096-A-06" {
                          }
                          frame "Custom" {
                          }
                        }
                        n2215 = Concatenate Strings("Test Standard :" ("Content"), w3265) -> (w3267:string)
                        n2216 = local read "EVENT LOG"() -> (w3270:string)
                        n2217 = call "Event Log.vi"("Content"=w3267, "EVENT LOG"=w3270) -> ("EVENT LOG"=w3269:string)  [unwired: 8 in, 1 out]
                        n2218 = local write "EVENT LOG"(w3269) -> ()
                      }
                      frame #12 {
                        n2219 = Wait (ms)(milliseconds to wait=u32 50) -> ()  [unwired: 1 out]
                      }
                      frame #13 {
                        n2220 = local read "Fuel Discription :"() -> (w3276:string)
                        n2221 = Concatenate Strings("Fuel Description :" ("Content"), w3276) -> (w3277:string)
                        n2222 = local read "EVENT LOG"() -> (w3280:string)
                        n2223 = call "Event Log.vi"("Content"=w3277, "EVENT LOG"=w3280) -> ("EVENT LOG"=w3279:string)  [unwired: 8 in, 1 out]
                        n2224 = local write "EVENT LOG"(w3279) -> ()
                      }
                      frame #14 {
                        n2225 = Wait (ms)(milliseconds to wait=u32 50) -> ()  [unwired: 1 out]
                      }
                      frame #15 {
                        n2226 = local read "Remarks :"() -> (w3282:string)
                        n2227 = Concatenate Strings("Remarks :" ("Content"), w3282) -> (w3283:string)
                        n2228 = local read "EVENT LOG"() -> (w3286:string)
                        n2229 = call "Event Log.vi"("Content"=w3283, "EVENT LOG"=w3286) -> ("EVENT LOG"=w3285:string)  [unwired: 8 in, 1 out]
                        n2230 = local write "EVENT LOG"(w3285) -> ()
                      }
                      frame #16 {
                        n2231 = Wait (ms)(milliseconds to wait=u32 50) -> ()  [unwired: 1 out]
                      }
                      frame #17 {
                        n2232 = local read "Operator ID"() -> (w3288:string)
                        n2233 = Concatenate Strings("Operator ID :" ("Content"), w3288) -> (w3290:string)
                        n2234 = local read "EVENT LOG"() -> (w3292:string)
                        n2235 = call "Event Log.vi"("Content"=w3290, "EVENT LOG"=w3292) -> ("EVENT LOG"=w3291:string)  [unwired: 8 in, 1 out]
                        n2236 = local write "EVENT LOG"(w3291) -> ()
                      }
                      frame #18 {
                        n2237 = Wait (ms)(milliseconds to wait=u32 50) -> ()  [unwired: 1 out]
                      }
                      frame #19 {
                        n2238 = disable-structure shown="Disabled" {
                          frame Disabled {
                            n2239 = local read "EVENT LOG"() -> (w3296:string)
                            n2240 = call "Event Log.vi"("Content"="Test Parameter", "EVENT LOG"=w3296) -> ("EVENT LOG"=w3295:string)  [unwired: 8 in, 1 out]
                            n2241 = local write "EVENT LOG"(w3295) -> ()
                          }
                          frame Enabled {
                          }
                        }
                      }
                      frame #20 {
                        n2242 = Wait (ms)(milliseconds to wait=u32 50) -> ()  [unwired: 1 out]
                      }
                      frame #21 {
                        n2243 = local read "Set Hz"() -> (w3300:dbl)
                        n2244 = Number To Fractional String(number=w3300, precision (6)=i16 2) -> (F-format string=w3299:string)  [unwired: 2 in]
                        n2245 = Concatenate Strings("Set Frequency [Hz] :" ("Content"), w3299) -> (w3302:string)
                        n2246 = local read "EVENT LOG"() -> (w3304:string)
                        n2247 = call "Event Log.vi"("Content"=w3302, "EVENT LOG"=w3304) -> ("EVENT LOG"=w3303:string)  [unwired: 8 in, 1 out]
                        n2248 = local write "EVENT LOG"(w3303) -> ()
                      }
                      frame #22 {
                        n2249 = Wait (ms)(milliseconds to wait=u32 50) -> ()  [unwired: 1 out]
                      }
                      frame #23 {
                        n2250 = local read "NORMAL LOAD"() -> (w3307:dbl)
                        n2251 = Number To Fractional String(number=w3307, precision (6)=i16 2) -> (F-format string=w3308:string)  [unwired: 2 in]
                        n2252 = Concatenate Strings("Applied Load [grams] :" ("Content"), w3308) -> (w3310:string)
                        n2253 = local read "EVENT LOG"() -> (w3312:string)
                        n2254 = call "Event Log.vi"("Content"=w3310, "EVENT LOG"=w3312) -> ("EVENT LOG"=w3311:string)  [unwired: 8 in, 1 out]
                        n2255 = local write "EVENT LOG"(w3311) -> ()
                      }
                      frame #24 {
                        n2256 = Wait (ms)(milliseconds to wait=u32 50) -> ()  [unwired: 1 out]
                      }
                      frame #25 {
                        n2257 = local read "Set Strk"() -> (w3315:dbl)
                        n2258 = Number To Fractional String(number=w3315, precision (6)=i16 2) -> (F-format string=w3316:string)  [unwired: 2 in]
                        n2259 = Concatenate Strings("Set Stroke [mm] :" ("Content"), w3316) -> (w3318:string)
                        n2260 = local read "EVENT LOG"() -> (w3320:string)
                        n2261 = call "Event Log.vi"("Content"=w3318, "EVENT LOG"=w3320) -> ("EVENT LOG"=w3319:string)  [unwired: 8 in, 1 out]
                        n2262 = local write "EVENT LOG"(w3319) -> ()
                      }
                      frame #26 {
                        n2263 = Wait (ms)(milliseconds to wait=u32 50) -> ()  [unwired: 1 out]
                      }
                      frame #27 {
                        n2264 = local read "Set Temp"() -> (w3323:dbl)
                        n2265 = Number To Fractional String(number=w3323, precision (6)=i16 2) -> (F-format string=w3324:string)  [unwired: 2 in]
                        n2266 = Concatenate Strings("Set Temperature [deg C] :" ("Content"), w3324) -> (w3326:string)
                        n2267 = local read "EVENT LOG"() -> (w3328:string)
                        n2268 = call "Event Log.vi"("Content"=w3326, "EVENT LOG"=w3328) -> ("EVENT LOG"=w3327:string)  [unwired: 8 in, 1 out]
                        n2269 = local write "EVENT LOG"(w3327) -> ()
                      }
                      frame #28 {
                        n2270 = Wait (ms)(milliseconds to wait=u32 50) -> ()  [unwired: 1 out]
                      }
                      frame #29 {
                        n2271 = local read "Set Rh"() -> (w3331:dbl)
                        n2272 = Number To Fractional String(number=w3331, precision (6)=i16 2) -> (F-format string=w3332:string)  [unwired: 2 in]
                        n2273 = Concatenate Strings("Set Humidity [%RH] :" ("Content"), w3332) -> (w3334:string)
                        n2274 = local read "EVENT LOG"() -> (w3336:string)
                        n2275 = call "Event Log.vi"("Content"=w3334, "EVENT LOG"=w3336) -> ("EVENT LOG"=w3335:string)  [unwired: 8 in, 1 out]
                        n2276 = local write "EVENT LOG"(w3335) -> ()
                      }
                      frame #30 {
                        n2277 = Wait (ms)(milliseconds to wait=u32 50) -> ()  [unwired: 1 out]
                      }
                      frame #31 {
                        n2278 = local read "test time"() -> (w3339:dbl)
                        n2279 = Number To Fractional String(number=w3339, precision (6)=i16 1) -> (F-format string=w3340:string)  [unwired: 2 in]
                        n2280 = Concatenate Strings("Test Duration [mins] :" ("Content"), w3340) -> (w3342:string)
                        n2281 = local read "EVENT LOG"() -> (w3344:string)
                        n2282 = call "Event Log.vi"("Content"=w3342, "EVENT LOG"=w3344) -> ("EVENT LOG"=w3343:string)  [unwired: 8 in, 1 out]
                        n2283 = local write "EVENT LOG"(w3343) -> ()
                      }
                      frame #32 {
                        w3345 = dbl[] [] ("History Data")
                        w3346 = cluster{"y":dbl, dbl, "y":dbl}[] [] ("History Data")
                        w3347 = FALSE ("Visible")
                        n2284 = property on="Stroke ( mm )" class="WFChart (strict)"("History Data"=w3346) -> ()  [unwired: 2 in, 2 out]
                        n2285 = property on="Humidity ( %RH )" class="WFChart (strict)"("History Data"=w3345) -> ()  [unwired: 2 in, 2 out]
                        n2286 = property on="Temperature ( Deg C )" class="WFChart (strict)"("History Data"=w3345) -> ()  [unwired: 2 in, 2 out]
                        n2287 = property on="Electrical Contact Resistance ( % )" class="WFChart (strict)"("History Data"=w3345) -> ()  [unwired: 2 in, 2 out]
                        n2288 = property on="Coefficient of Friction" class="WFChart (strict)"("History Data"=w3345) -> ()  [unwired: 2 in, 2 out]
